vi "Process.vi"(8 "error in (no error)":errorcluster, 11 "Generic Handler in":refnum<class "Generic Handler.lvclass">) -> (0 "error out":errorcluster, 3 "Generic Handler out":refnum<class "Generic Handler.lvclass">)   [LabVIEW 2025, in "Generic Handler.lvclass"]
uses:
  Generic Handler.lvclass
  <vilib>/Handler Framework/Handler/Handler.lvclass
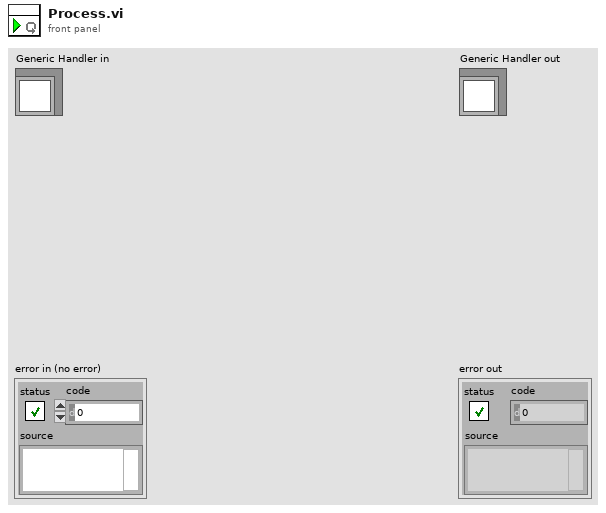
[diagram p1: front panel]
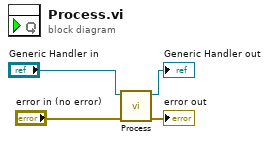
[diagram p0: block diagram]
diagram:
  n1 = call-parent "Process.vi"("error in (no error)"="error in (no error)", "Handler in"="Generic Handler in") -> ("error out"=→"error out":errorcluster, "Handler out"=→"Generic Handler out":refnum<class "Generic Handler.lvclass">)  [unwired: 8 in]
